vi "xy-pi-control.vi"(5 "Ki-xy":sgl=0.001 format="%#_13g", 7 "xy-umax":sgl, 8 "xy-ref":sgl[](array[numeric])=[0.0, 0.0], 11 "x_k-y_k":fxp<+/-,25,6>[](array[numeric])=[0.0, 0.0]) -> (0 "u_y saturated":bool, 1 "u_x saturated":bool, 2 "sat(u_y)":sgl, 3 "sat(u_x)":sgl)   [LabVIEW 2017]
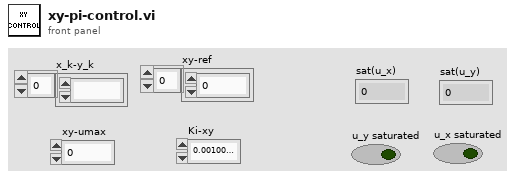
[diagram p1: front panel]
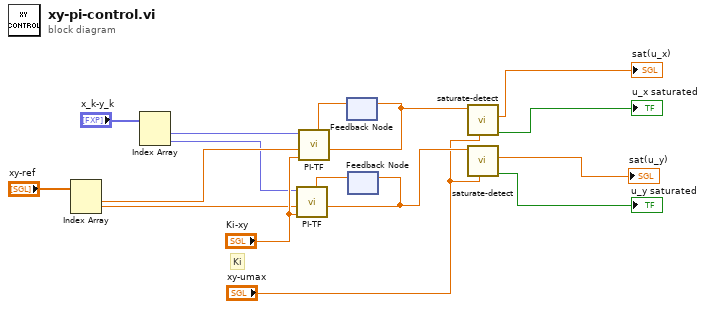
[diagram p0: block diagram]
diagram:
  # "Ki"
  n1 = Index Array(array="xy-ref") -> (element #1=w6:sgl, element #2=w5:sgl)  [unwired: 2 in]
  n2 = Index Array(array="x_k-y_k") -> (element #1=w3:fxp<+/-,25,6>, element #2=w2:fxp<+/-,25,6>)  [unwired: 2 in]
  n3 = feedback #1() -> (w9:sgl)  [unwired: 1 in]
  n4 = call "PI-TF.vi"("u(k-1)"=w9, "Ki"="Ki-xy", "setpoint"=w6, "y(k)"=w3) -> ("u(k)"=w14:sgl)  [unwired: 7 in]
  n5 = feedback-in #1(w14) -> ()
  n6 = feedback #2() -> (w10:sgl)  [unwired: 1 in]
  n7 = call "PI-TF.vi"("u(k-1)"=w10, "Ki"="Ki-xy", "setpoint"=w5, "y(k)"=w2) -> ("u(k)"=w13:sgl)  [unwired: 7 in]
  n8 = feedback-in #2(w13) -> ()
  n9 = call "saturate-detect.vi"("bound"="xy-umax", "x"=w14) -> ("saturated"=→"u_x saturated":bool, "sat(x)"=→"sat(u_x)":sgl)  [unwired: 8 in]
  n10 = call "saturate-detect.vi"("bound"="xy-umax", "x"=w13) -> ("saturated"=→"u_y saturated":bool, "sat(x)"=→"sat(u_y)":sgl)  [unwired: 8 in]
